vi "Generate Random String.vi"(4 "String Length (5)":i32=5) -> (1 "Output String":string)   [LabVIEW 2011]
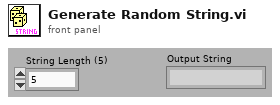
[diagram p1: front panel]
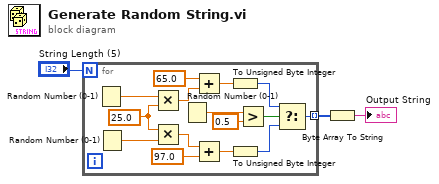
[diagram p0: block diagram]
diagram:
  n1 = for {
    N: "String Length (5)" -> [_]
    tunnel: [w4] -> w2 mode=indexing
    w11 = 25.0 ("x")
    n2 = Random Number (0-1)() -> (number: 0 to 1=w10:dbl)
    n3 = Random Number (0-1)() -> (number: 0 to 1=w12:dbl)
    n4 = Multiply(x=w10, y=w11) -> (x*y=w13:dbl)
    n5 = Multiply(x=w11, y=w12) -> (x*y=w14:dbl)
    n6 = Random Number (0-1)() -> (number: 0 to 1=w9:dbl)
    n7 = Add(x=65.0, y=w13) -> (x+y=w18:dbl)
    n8 = Add(x=w14, y=97.0 ("x")) -> (x+y=w15:dbl)
    n9 = To Unsigned Byte Integer(number=w18) -> (unsigned 8bit integer=w6:u8)
    n10 = To Unsigned Byte Integer(number=w15) -> (unsigned 8bit integer=w5:u8)
    n11 = Greater?(x=w9, y=0.5) -> (0:w7:bool)
    n12 = Select(t=w6, s=w7, f=w5) -> (s? t:f=w4:u8)
  }
  n13 = Byte Array To String(unsigned byte array=w2) -> (string=→"Output String":string)
